vi "FrecMod%.vi"(9 "iteracion":i32, 11 "Frec Input":sgl) -> (0 "cada 10 seg":bool, 1 "alarma":bool, 3 "Frecuency Modulation (%)":sgl)   [LabVIEW 2018]
doc: "[Ver 1.00]\n\nDESCRIPCION\nSaca el promedio de las últimas 10 mediciones, que equivalen a 10 segundos de medicion y hace el cálculo de Tolerancia en la Modulación, según la IEEE45.\n\nLIMITES = 0,5%"
panel:
  out "size(s)":i32
  # "Input"
  # "Local"
  # "Output"
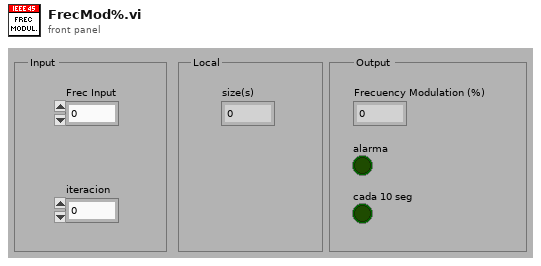
[diagram p1: front panel]
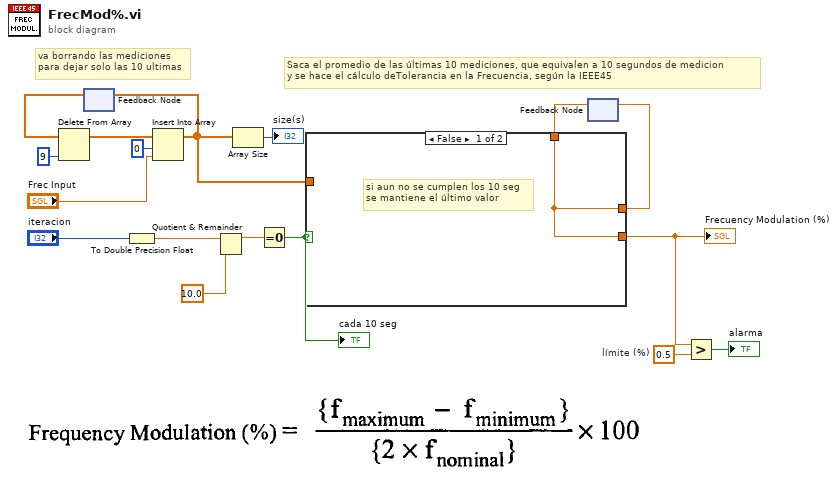
[diagram p0: block diagram]
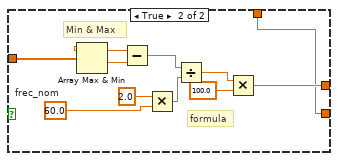
[diagram p2: hidden frame]
diagram:
  w3 = sgl 0.5  # límite (%)
  # "va borrando las mediciones\npara dejar solo las 10 ultimas"
  # "Saca el promedio de las últimas 10 mediciones, que equivalen a 10 segundos de medicion\ny se hace el cálculo deTolerancia en la Frecuencia, según la IEEE45"
  n1 = feedback #1() -> (w17:sgl[])  [unwired: 1 in]
  n2 = Delete From Array(array=w17, index=9) -> (array with subset deleted=w14:sgl[])  [unwired: 1 in, 1 out]
  n3 = To Double Precision Float(number="iteracion") -> (double precision float=w4:dbl)
  n4 = Insert Into Array(array=w14, index=0, new element="Frec Input") -> (w10:sgl[])
  n5 = feedback-in #1(w10) -> ()
  n6 = Quotient & Remainder(x=w4, y=10.0) -> (x-y*floor(x/y)=w11:dbl)  [unwired: 1 out]
  n7 = Array Size(array=w10) -> (size(s)=→"size(s)":i32)
  n8 = Equal To 0?(x=w11) -> (x = 0?=w9:bool)
  "cada 10 seg" <- w9
  n9 = feedback #2() -> (w5:sgl)  [unwired: 1 in]
  n10 = case shown="False" w9 {
    tunnel: w10 -> [_ w29]
    tunnel: [w18 w20] -> w6
    tunnel: [w18 w19] -> w2
    tunnel: w5 -> [w18 w19]
    frame False {
      # "si aun no se cumplen los 10 seg\nse mantiene el último valor"
    }
    frame True {
      w25 = sgl 60.0  # frec_nom
      # "Min & Max"
      # "formula"
      n11 = Array Max & Min(array=w29) -> (max value=w28:sgl, min value=w27:sgl)  [unwired: 2 out]
      n12 = Subtract(x=w28, y=w27) -> (x-y=w23:sgl)
      n13 = Multiply(x=sgl 2.0, y=w25) -> (x*y=w24:sgl)
      n14 = Divide(x=w23, y=w24) -> (x/y=w22:sgl)
      n15 = Multiply(x=w22, y=sgl 100.0) -> (x*y=w20:sgl)
    }
  }
  "Frecuency Modulation (%)" <- w2
  n16 = feedback-in #2(w6) -> ()
  n17 = Greater?(x=w2, y=w3) -> (0:→"alarma":bool)
